vi "GDI_Resize.vi"(7 "filename":path, 8 "error in (no error)":errorcluster, 9 "old image":picture, 10 "height":i16=400, 11 "width":i16=800) -> (0 "error out":errorcluster, 3 "new picture":picture)   [LabVIEW 2020, in "GraphBG_manage.lvlib" / "Graph.lvclass"]
uses:
  Graph.lvclass
  <vilib>/Utility/miscctls.llb/LVBoundsTypeDef.ctl
  System.Drawing
  <vilib>/wsapi/NI_WebServices.lvlib
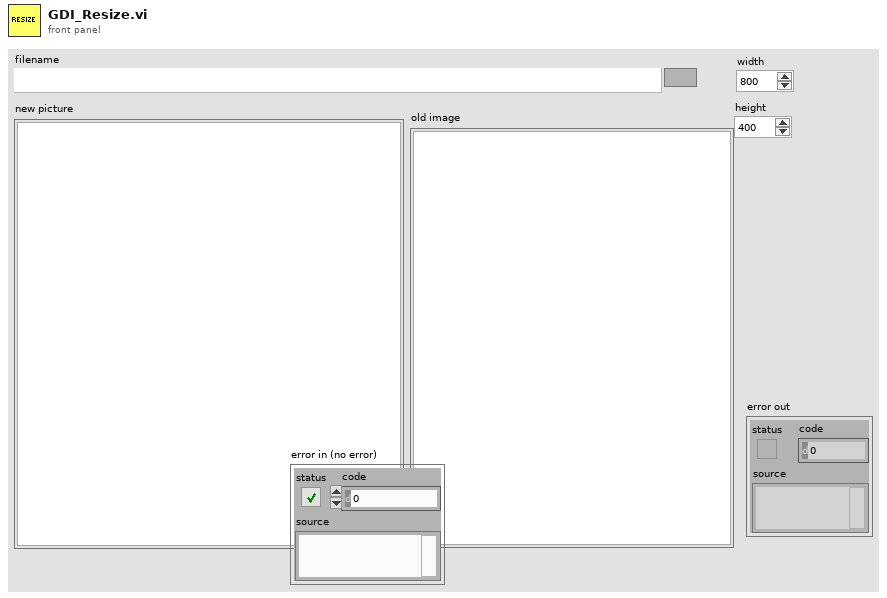
[diagram p1: front panel]
types:
  T1 = typedef "LVBoundsTypeDef.ctl" = cluster{"Width":u32, "Height":u32}
  T2 = typedef "imagedata.ctl" = cluster{"image type":i32, "image depth":i32, "image":u8[], "mask":u8[], "colors":u32[], "Rectangle":cluster{"left":i16, "top":i16, "right":i16, "bottom":i16}}
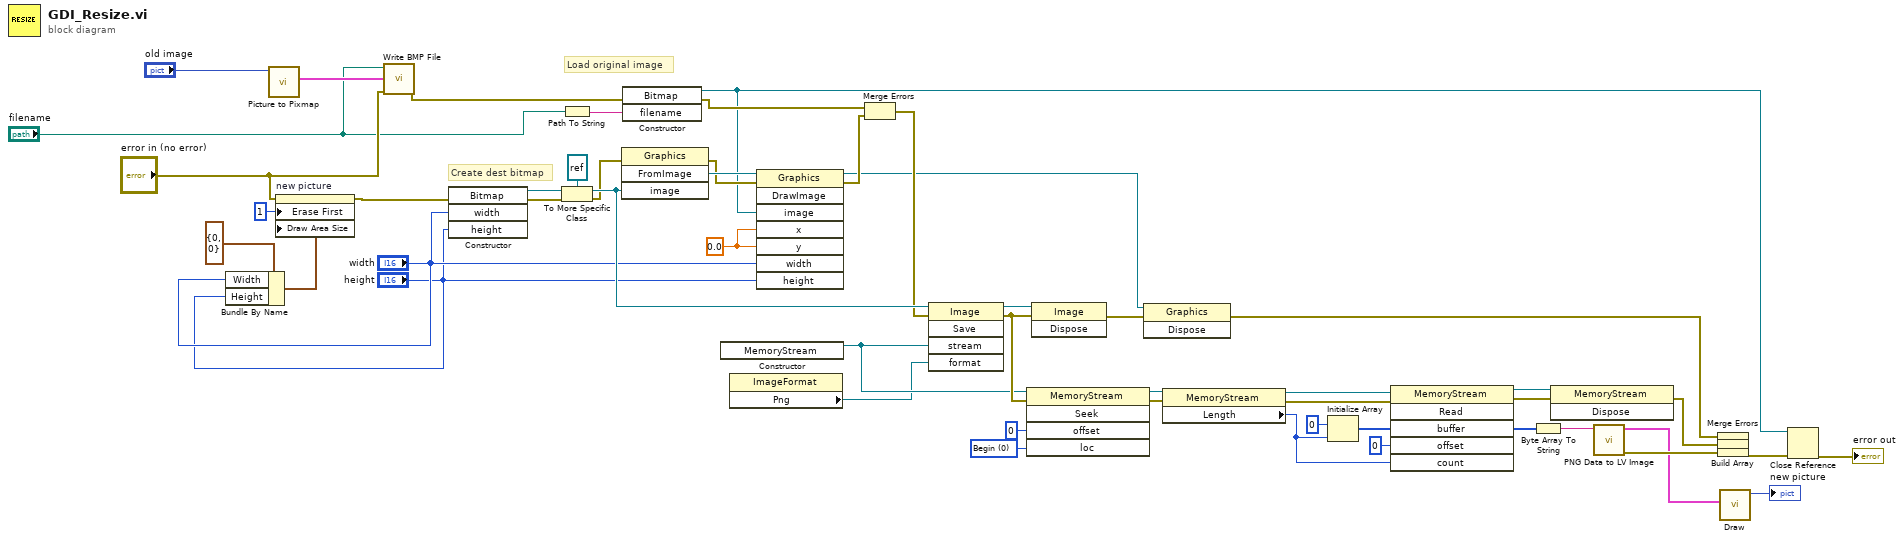
[diagram p0: block diagram]
diagram:
  w44 = 0 items=["Begin", "Current", "End"] ("loc")
  w52 = sgl 0.0 ("x")
  # "Create dest bitmap"
  # "Load original image"
  n1 = Bundle By Name(cluster=T1 {"Width"=0, "Height"=0} ("Draw Area Size"), "Width"="width", "Height"="height") -> (w18:T1)
  n2 = call <vilib>:"Picture to Pixmap.vi"("picture"="old image") -> ("image data"=w11:T2)  [unwired: 9 in, 1 out]
  n3 = property on="new picture" class="Pict"(error in="error in (no error)", "Erase First"=u8 1, "Draw Area Size"=w18) -> (error out=w17:errorcluster)  [unwired: 1 in, 1 out]
  n4 = call <vilib>:"Write BMP File.vi"("error in (no error)"="error in (no error)", "image data"=w11, "path to BMP file"="filename") -> ("error out"=w13:errorcluster)  [unwired: 7 in, 1 out]
  n5 = constructor class="Bitmap"(error in=w17, "width"="width", "height"="height") -> (reference out=w50:refnum<k24>, error out=w28:errorcluster)  [unwired: 2 in, 3 out]
  n6 = Path To String(path="filename") -> (string=w4:string)
  n7 = To More Specific Class(target class=refnum<k24> refnum, reference=w50, error in=w28) -> (specific class reference=w32:refnum<k24>, error out=w27:errorcluster)
  n8 = invoke class="Graphics" method="FromImage"(error in=w27, "image"=w32) -> (error out=w26:errorcluster, "FromImage"=w49:refnum<k24>)  [unwired: 2 in, 2 out]
  n9 = constructor class="Bitmap"(error in=w13, "filename"=w4) -> (reference out=w3:refnum<k24>, error out=w10:errorcluster)  [unwired: 2 in, 2 out]
  n10 = constructor class="MemoryStream"() -> (reference out=w23:refnum<k24>)  [unwired: 3 in, 2 out]
  n11 = property class="ImageFormat"() -> ("Png"=w22:refnum<k24>)  [unwired: 2 in, 2 out]
  n12 = invoke class="Graphics" method="DrawImage"(reference=w49, error in=w26, "image"=w3, "x"=w52, "y"=w52, "width"="width", "height"="height") -> (reference out=w6:refnum<k24>, error out=w25:errorcluster)  [unwired: 1 in, 6 out]
  n13 = Merge Errors(w10, w25) -> (w24:errorcluster)
  n14 = invoke class="Image" method="Save"(reference=w32, error in=w24, "stream"=w23, "format"=w22) -> (reference out=w48:refnum<k24>, error out=w35:errorcluster)  [unwired: 1 in, 3 out]
  n15 = invoke class="MemoryStream" method="Seek"(reference=w23, error in=w35, "offset"=i64 0, "loc"=w44) -> (reference out=w47:refnum<k24>, error out=w46:errorcluster)  [unwired: 1 in, 3 out]
  n16 = invoke class="Image" method="Dispose"(reference=w48, error in=w35) -> (error out=w7:errorcluster)  [unwired: 1 in, 2 out]
  n17 = invoke class="Graphics" method="Dispose"(reference=w6, error in=w7) -> (error out=w5:errorcluster)  [unwired: 1 in, 2 out]
  n18 = property class="MemoryStream"(reference=w47, error in=w46) -> (reference out=w42:refnum<k24>, error out=w41:errorcluster, "Length"=w39:i64)
  n19 = Initialize Array(u8 0 ("element"), w39) -> (w40:u8[])
  n20 = invoke class="MemoryStream" method="Read"(reference=w42, error in=w41, "buffer"=w40, "offset"=0, "count"=w39) -> (reference out=w37:refnum<k24>, error out=w36:errorcluster, "buffer"=w34:u8[])  [unwired: 1 in, 3 out]
  n21 = Byte Array To String(unsigned byte array=w34) -> (string=w31:string)
  n22 = invoke class="MemoryStream" method="Dispose"(reference=w37, error in=w36) -> (error out=w33:errorcluster)  [unwired: 1 in, 2 out]
  n23 = call <vilib>:"PNG Data to LV Image.vi"("png data"=w31) -> ("error out"=w30:errorcluster, "image data"=w21:T2)  [unwired: 9 in]
  n24 = Build Array(w5, w33, w30) -> (w29:errorcluster[])
  n25 = Merge Errors(w29) -> (w9:errorcluster)
  n26 = call "Draw.vi"("image data"=w21) -> ("new picture"=→"new picture":picture)  [unwired: 8 in]
  n27 = Close Reference(reference=w3, error in (no error)=w9) -> (error out=→"error out":errorcluster)
